vi "RSZVB Get Calibration Data Parameters.vi"(0 "VISA session":refnum<visa-resource-name>, 5 "Channel (1)":i32=1, 11 "error in (no error)":errorcluster {"code" format="%.0x"}) -> (3 "Frequency Start":dbl format="%^.3e", 4 "dup VISA session":refnum<visa-resource-name>, 6 "Frequency Stop":dbl format="%^.3e", 8 "Number Of Points":i32, 10 "Internal Signal Source Power":dbl format="%^.3e", 14 "Sweep Type":i32, 15 "error out":errorcluster {"code" format="%.0x"})   [LabVIEW 2011]
doc: "This VI queries the parameters of the channel's calibration\n\nRemote-control command(s):\n[SENSe<Ch>:]CORRection:DATA:PARameter?"
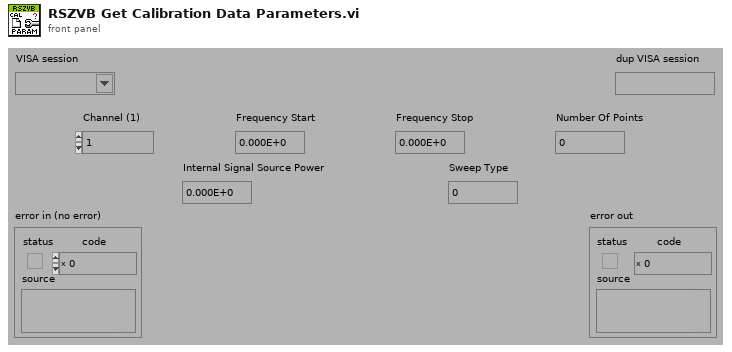
[diagram p1: front panel]
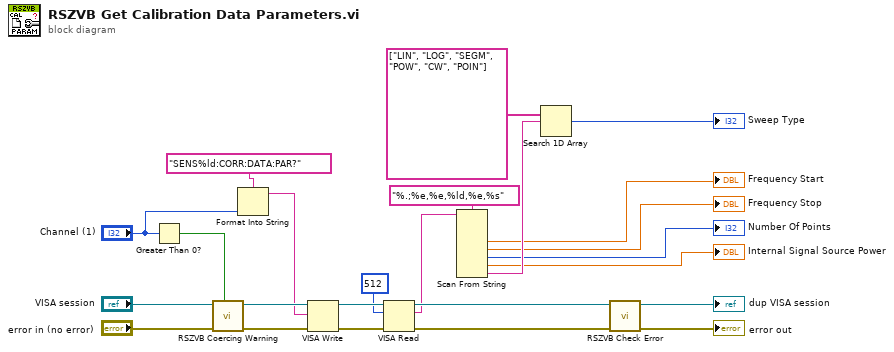
[diagram p0: block diagram]
diagram:
  n1 = Greater Than 0?(x="Channel (1)") -> (x > 0?=w17:bool)
  n2 = call "RSZVB Coercing Warning.vi"("In Range?"=w17, "error in (no error)"="error in (no error)", "VISA session"="VISA session") -> ("error out"=w22:errorcluster, "dup VISA session"=w23:refnum<visa-resource-name>)  [unwired: 7 in]
  n3 = Format Into String(format string="SENS%ld:CORR:DATA:PAR?", "Channel (1)") -> (resulting string=w14:string)  [unwired: 2 in, 1 out]
  n4 = VISA Write(VISA resource name=w23, write buffer=w14, error in (no error)=w22) -> (VISA resource name out=w21:refnum<visa-resource-name>, error out=w20:errorcluster)  [unwired: 1 out]
  n5 = VISA Read(VISA resource name=w21, byte count=u32 512 ("byte count (0)"), error in (no error)=w20) -> (VISA resource name out=w19:refnum<visa-resource-name>, read buffer=w12:string, error out=w18:errorcluster)  [unwired: 1 out]
  n6 = Scan From String(format string="%.;%e,%e,%ld,%e,%s", input string=w12) -> (output 1=→"Frequency Start":dbl, output 2=→"Frequency Stop":dbl, output 3=→"Number Of Points":i32, output 4=→"Internal Signal Source Power":dbl, output 5=w6:string)  [unwired: 7 in, 3 out]
  n7 = Search 1D Array(1D array=string[] ["LIN", "LOG", "SEGM", "POW", "CW", "POIN"], element=w6) -> (index of element=→"Sweep Type":i32)  [unwired: 1 in]
  n8 = call "RSZVB Check Error.vi"("error in (no error)"=w18, "VISA session"=w19) -> ("error out"=→"error out":errorcluster, "dup VISA session"=→"dup VISA session":refnum<visa-resource-name>)  [unwired: 8 in]
